vi "Constants.vi"() -> ()   [LabVIEW 2019, in "HLA Custom Device Shared.lvlib"]
doc: "Use this Global VI to access the GUIDs assigned to the page resources of the Custom Device."
uses:
  HLA Custom Device Configuration.llb/HLA Custom Device Shared.lvlib
panel:
  in  "Tab Control":enum32{"GUIDs", "Constants", "Properties"}(tab)
  in  "Parameter":string="b77a7904-c8be-44c8-af97-10fb8448d551"
  in  "Attribute":string="cf0d2834-1ef6-435c-a08f-d62632844e08"
  in  "Interaction":string="53780803-8140-4f62-8208-f49394e419e9"
  in  "Object":string="52d4cd88-974f-4360-a8ff-7bc610057bee"
  in  "FOM":string="8562ebb4-606d-4f7b-bdb0-39fb194478f7"
  in  "HLA Custom Device":string="6f4b2c5e-9a04-4726-97a9-de47f61042c2"
  in  "Compiled.Settings":string="Compiled.Settings"
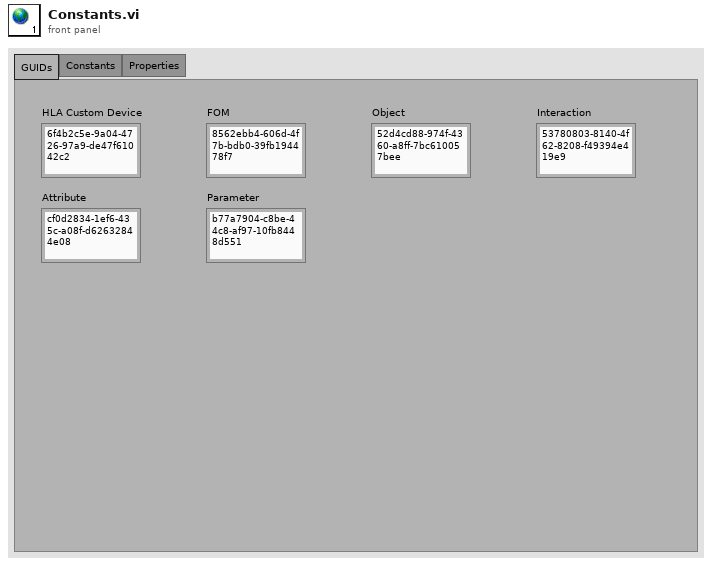
[diagram p1: front panel]
diagram:
